vi "is labview running.vi"(8 "error in":errorcluster) -> (0 "error out":errorcluster, 3 "running":bool)   [LabVIEW 2013]
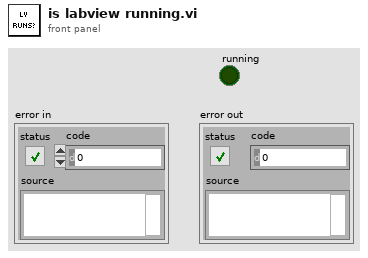
[diagram p1: front panel]
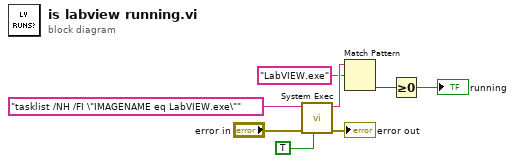
[diagram p0: block diagram]
diagram:
  n1 = call <vilib>:"System Exec.vi"("run minimized? (F)"=TRUE, "error in (no error)"="error in", "command line"="tasklist /NH /FI \"IMAGENAME eq LabVIEW.exe\"") -> ("error out"=→"error out":errorcluster, "standard output"=w3:string)  [unwired: 5 in, 2 out]
  n2 = Match Pattern(string=w3, regular expression="LabVIEW.exe" ("search string")) -> (offset past match=w1:i32)  [unwired: 1 in, 3 out]
  n3 = Greater Or Equal To 0?(x=w1) -> (x >= 0?=→"running":bool)
